vi "Test check.vi"() -> ()   [LabVIEW 2014]
uses:
  AISAS motor.lvclass
panel:
  in  "stop":bool
  out "Sync response":string
  out "AISAS motors ok?":bool[](array[boolean])
  out "error out":errorcluster
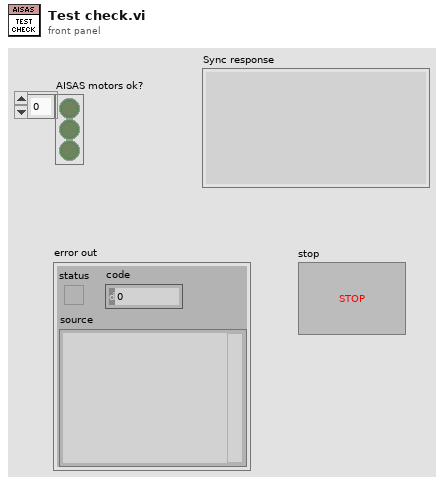
[diagram p1: front panel]
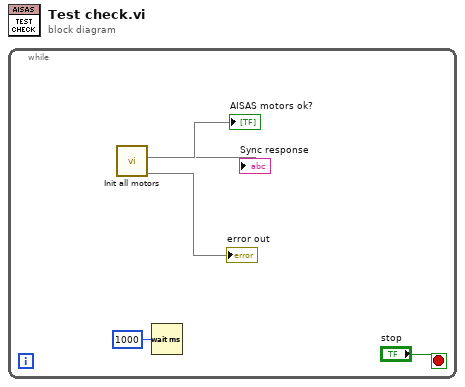
[diagram p0: block diagram]
diagram:
  n1 = while {
    stop <- "stop" stop-if-true
    n2 = call "Init all motors.vi"() -> (0:→"error out", 1:→"Sync response", 2:→"AISAS motors ok?")  [unwired: 8 in, 1 out]
    n3 = Wait (ms)(milliseconds to wait=u32 1000 ("millisecond multiple")) -> ()  [unwired: 1 out]
  }
